vi "Discrete Transfer Function (DBL Array).vi"(2 "initialize":bool, 3 "transfer functions":T1(array[cluster])=[{"numerator"=[], "denominator"=[]}] {"denominator" format="%.2f"; "numerator" format="%.2f"}, 5 "input points":dbl[](array[numeric]) format="%.2f") -> (1 "output points":dbl[](array[numeric]) format="%.2f")   [LabVIEW 2017, in "NI_AdvCtrl_discrete linear.lvlib"]
doc: "LabVIEW no longer supports this VI. You can obtain similar functionality by installing the LabVIEW Simulation Module.\n\nCalculates a new output, where the transfer function (numerator and denominator polynomials) and the input are given. It is H(z)=Numerator(z)/Denominator(z)."
uses:
  <vilib>/addons/control/advanced/NI_AdvCtrl_discrete linear.lvlib
  <vilib>/addons/control/advanced/NI_AdvCtrl_continuous linear.lvlib
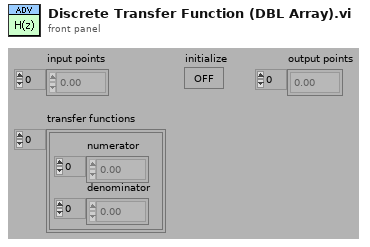
[diagram p1: front panel]
types:
  T1 = cluster{"numerator":dbl[], "denominator":dbl[]}[]
  T2 = cluster{"Numerator new":dbl[], "Denominator new":dbl[]}[]
  T3 = cluster{"Numerator new":dbl[], "Denominator new":dbl[]}
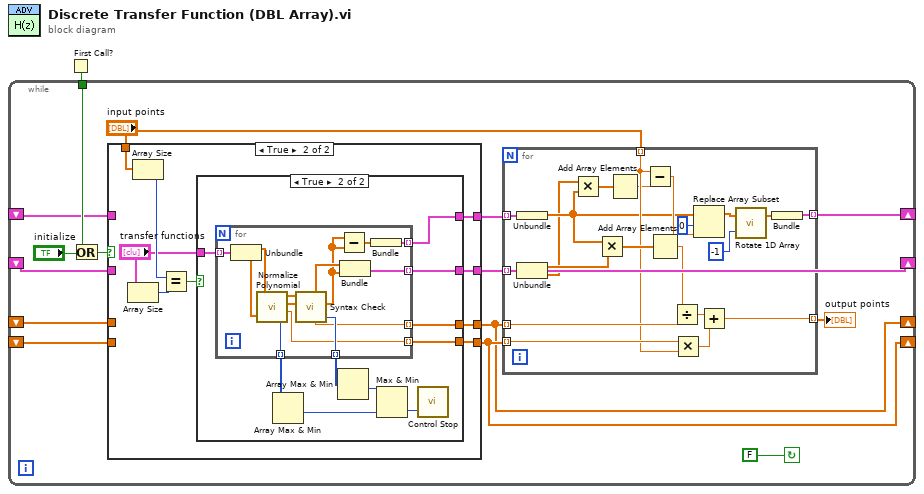
[diagram p0: block diagram]
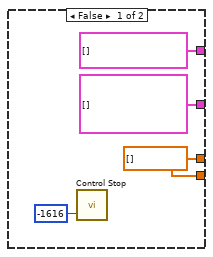
[diagram p3: hidden frame]
diagram:
  n1 = First Call?() -> (First Call?: T/F=w1:bool)
  n2 = while {
    shift-left: _ -> [w4]
    shift-right: [w5] -> _
    shift-left: _ -> [w7]
    shift-right: [w8] -> _
    tunnel: w1 -> [w10]
    shift-left: _ -> [w15]
    shift-right: [w14] -> _
    shift-left: _ -> [w16]
    shift-right: [w13] -> _
    stop <- FALSE continue-if-true
    n3 = Or(x=w10, y="initialize") -> (x .or. y?=w9:bool)
    n4 = case shown="True" w9 {
      tunnel: [w40 w50] -> w14
      tunnel: [w41 w49] -> w13
      tunnel: w16 -> [w41 _]
      tunnel: w15 -> [w40 _]
      tunnel: w7 -> [w38 _]
      tunnel: [w39 w48] -> w5
      tunnel: [w38 w46] -> w3
      tunnel: w4 -> [w39 _]
      tunnel: "input points" -> [_ w47]
      frame False {
      }
      frame True {
        n5 = Array Size(array="transfer functions") -> (size(s)=w44:i32)
        n6 = Array Size(array=w47) -> (size(s)=w45:i32)
        n7 = Equal?(x=w45, y=w44) -> (x = y?=w42:bool)
        n8 = case shown="True" w42 {
          tunnel: [w52 w64] -> w50
          tunnel: [w52 w63] -> w49
          tunnel: "transfer functions" -> [_ w62]
          tunnel: [T2 [] w61] -> w48
          tunnel: [cluster{dbl[]}[] [] w55] -> w46
          frame False {
            w52 = dbl[] []
            n9 = call <vilib>:"Control Stop.vi"("error"=-1616) -> ()  [unwired: 2 out]
          }
          frame True {
            n10 = for {
              tunnel: [w78] -> w60 mode=indexing
              tunnel: [w77] -> w59 mode=indexing
              tunnel: [w74] -> w64 mode=indexing
              tunnel: [w73] -> w63 mode=indexing
              tunnel: w62 -> [w72] mode=indexing
              tunnel: [w69] -> w61 mode=indexing
              tunnel: [w65] -> w55 mode=indexing
              n11 = Unbundle(w72) -> ("numerator"=w71:dbl[], "denominator"=w70:dbl[])
              n12 = call <vilib>:"Normalize Polynomial.vi"("Numerator"=w71, "Denominator"=w70) -> ("Numerator new"=w75:dbl[], "Denominator new"=w76:dbl[], "additive constant"=w74:dbl, "error"=w77:i32)
              n13 = call <vilib>:"Syntax Check.vi"("Denominator"=w76, "Numerator"=w75) -> ("error"=w78:i32, "gain"=w73:dbl, "Denominator new"=w67:dbl[], "Numerator new"=w68:dbl[])  [unwired: 1 out]
              n14 = Subtract(x=w67, y=w67) -> (x-y=w66:dbl[])
              n15 = Bundle("Numerator new"=w68, "Denominator new"=w67) -> (w69:T3)  [unwired: 1 out]
              n16 = Bundle(w66) -> (w65:cluster{dbl[]})  [unwired: 1 in]
            }
            n17 = Array Max & Min(array=w59) -> (min value=w57:i32)  [unwired: 3 out]
            n18 = Array Max & Min(array=w60) -> (min value=w58:i32)  [unwired: 3 out]
            n19 = Max & Min(x=w58, y=w57) -> (min(x,y)=w56:i32)  [unwired: 1 out]
            n20 = call <vilib>:"Control Stop.vi"("error"=w56) -> ()  [unwired: 2 out]
          }
        }
      }
    }
    n21 = for {
      tunnel: w14 -> [w35] mode=indexing
      tunnel: w13 -> [w34] mode=indexing
      tunnel: [w20] -> w8 mode=indexing
      tunnel: w3 -> [w27] mode=indexing
      tunnel: "input points" -> [w30] mode=indexing
      tunnel: [w29] -> w6 mode=indexing
      tunnel: w5 -> [w24] mode=indexing
      n22 = Unbundle(w27) -> ("array (last n elements first)"=w22:dbl[])
      n23 = Unbundle(w24) -> ("Numerator new"=w23:dbl[], "Denominator new"=w21:dbl[])
      n24 = Multiply(x=w21, y=w22) -> (x*y=w26:dbl[])
      n25 = Multiply(x=w22, y=w23) -> (x*y=w32:dbl[])
      n26 = Add Array Elements(numeric array=w26) -> (sum=w25:dbl)
      n27 = Subtract(x=w30, y=w25) -> (x-y=w33:dbl)
      n28 = Add Array Elements(numeric array=w32) -> (sum=w31:dbl)
      n29 = Divide(x=w31, y=w34) -> (x/y=w36:dbl)
      n30 = Multiply(x=w35, y=w30) -> (x*y=w37:dbl)
      n31 = Replace Array Subset(array=w22, new element=w33, index=0 ("Index")) -> (w18:dbl[])
      n32 = Add(x=w36, y=w37) -> (x+y=w29:dbl)
      n33 = call <vilib>:"Rotate 1D Array.vi"("n"=-1, "array"=w18) -> ("array (last n elements first)"=w19:dbl[])  [unwired: 1 out]
      n34 = Bundle("array (last n elements first)"=w19) -> (w20:cluster{"array (last n elements first)":dbl[]})  [unwired: 1 in]
    }
    "output points" <- w6
  }
